vi "MCP - custom error handler.vi"(7 "message":string, 8 "error in":errorcluster, 9 "call chain":string[](array[string]), 10 "Is Error?":bool=TRUE caption="Is Error? (def: TRUE)", 11 "custom error code":i32) -> (0 "error out":errorcluster)   [LabVIEW 2026, in "MicroPulse_Driver.lvlib"]
uses:
  MicroPulse_Driver.lvlib
  <vilib>/Utility/error.llb/DialogType.ctl
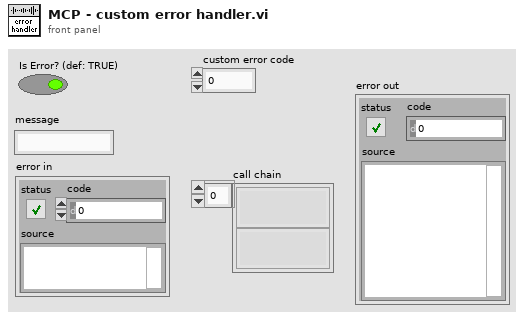
[diagram p1: front panel]
types:
  T1 = typedef "DialogType.ctl" = u16
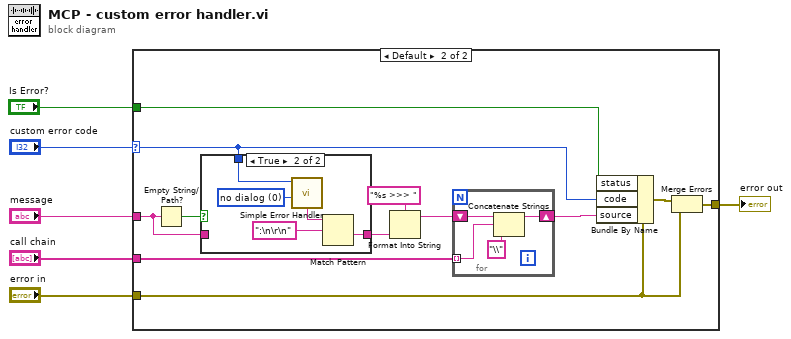
[diagram p0: block diagram]
diagram:
  n1 = case shown="Default" "custom error code" {
    selector: "custom error code" -> [_ w9]
    tunnel: "error in" -> [w7 w19]
    tunnel: "call chain" -> [_ w18]
    tunnel: "message" -> [_ w15]
    tunnel: [w7 w14] -> w3
    tunnel: "Is Error?" -> [_ w8]
    frame 0 {
    }
    frame Default {
      n2 = Empty String/Path?(string/path=w15) -> (empty?=w16:bool)
      n3 = case shown="True" w16 {
        tunnel: w15 -> [w20 _]
        tunnel: [w20 w25] -> w11
        tunnel: w9 -> [_ w21]
        frame False {
        }
        frame True {
          w23 = T1 0 items=["no dialog", "OK message", "continue or stop message", "OK message + warnings", "continue/stop + warnings"] ("type of dialog (OK msg:1)")
          n4 = call <vilib>:"Simple Error Handler.vi"("error code (no error:0)"=w21, "type of dialog (OK msg:1)"=w23) -> ("message"=w22:string)  [unwired: 3 in, 4 out]
          n5 = Match Pattern(string=w22, regular expression=":\n\r\n") -> (after substring=w25:string)  [unwired: 1 in, 3 out]
        }
      }
      n6 = Format Into String(format string="%s >>> ", w11) -> (resulting string=w10:string)  [unwired: 2 in, 1 out]
      n7 = for {
        tunnel: w18 -> [w29] mode=indexing
        shift-right: [w27] -> w17
        shift-left: w10 -> [w26]
        n8 = Concatenate Strings(w26, w29, "\\" ("format string")) -> (w27:string)
      }
      n9 = Bundle By Name(cluster=w19, "status"=w8, "code"=w9, "source"=w17) -> (w13:errorcluster)
      n10 = Merge Errors(w13, w19) -> (w14:errorcluster)
    }
  }
  "error out" <- w3
